vi "Waveform to CSV Converter.vi"(8 "error in (no error)":errorcluster, 11 "Waveform File Path (.wfm)":path) -> (0 "error out":errorcluster)   [LabVIEW 2013]
uses:
  <vilib>/Waveform/WDTFileIO.llb/Export Waveforms To Spreadsheet File (2D).vi
panel:
  out "Done":bool
  out "Zipping":bool
  out "Converting":bool
  out "Records read":i32
  # "Waveform to CSV Converter"
  # "This VI reads the Waveform data from the specified path and then writes all records to a CSV file.\nThis file is then added to a new Zip file and then deleted. The names of the CSV and Zip file are\nthe same as the Waveform file except with .wfm replaced with .csv and .zip respectively."
  # "27 Feb 2015\nby P. Lane"
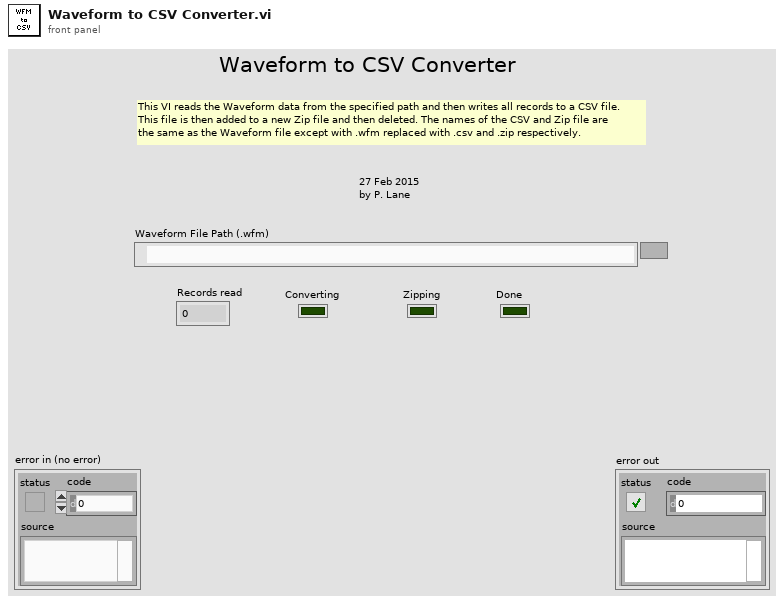
[diagram p1: front panel]
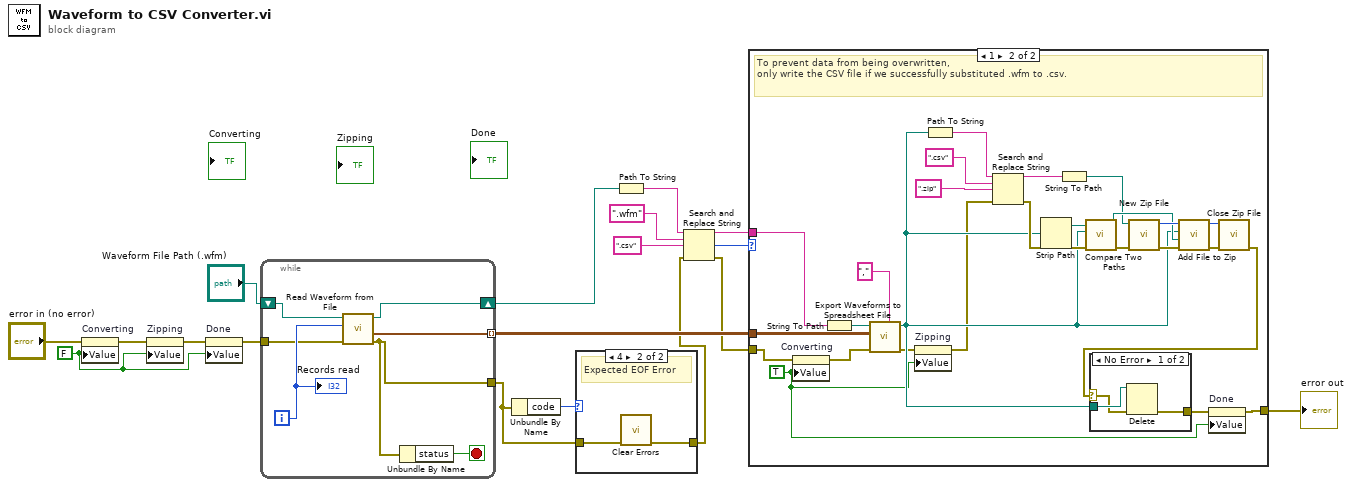
[diagram p0: block diagram]
diagram:
  w1 = FALSE ("Converted")
  n1 = property on="Converting" class="Bool (strict)"(error in="error in (no error)", "Value"=w1) -> (error out=w5:errorcluster)  [unwired: 1 in, 1 out]
  n2 = property on="Zipping" class="Bool (strict)"(error in=w5, "Value"=w1) -> (error out=w3:errorcluster)  [unwired: 1 in, 1 out]
  n3 = property on="Done" class="Bool (strict)"(error in=w3, "Value"=w1) -> (error out=w2:errorcluster)  [unwired: 1 in, 1 out]
  n4 = while {
    tunnel: [w23] -> w17 mode=indexing
    shift-right: [w22] -> w13
    shift-left: "Waveform File Path (.wfm)" -> [w21]
    tunnel: w2 -> [w20]
    tunnel: [w19] -> w9
    i -> [w25]
    stop <- w24 stop-if-true
    n5 = call <vilib>:"Read Waveform from File.vi"("error in (no error)"=w20, "offset (records:0)"=w25, "file path (dialog if empty)"=w21) -> ("error out"=w19:errorcluster, "all waveforms in record"=w23:waveform(dbl)[], "new file path (Not A Path if cancelled)"=w22:path)  [unwired: 3 in, 1 out]
    n6 = Unbundle By Name(w19) -> ("status"=w24:bool)
    "Records read" <- w25
  }
  n7 = Unbundle By Name(w9) -> ("code"=w10:i32)
  n8 = case shown="4" w10 {
    tunnel: w9 -> [w26 w28]
    tunnel: [w26 w27] -> w7
    frame 0, Default {
      # "Unexpected Error"
    }
    frame 4 {
      # "Expected EOF Error"
      n9 = call <vilib>:"Clear Errors.vi"("error in (no error)"=w28) -> ("error out"=w27:errorcluster)  [unwired: 6 in]
    }
  }
  n10 = Path To String(path=w13) -> (string=w14:string)
  n11 = Search and Replace String(input string=w14, search string=".wfm", replace string=".csv" ("replace string (\"\")"), error in=w7) -> (result string=w12:string, number of replacements=w11:i32, error out=w6:errorcluster)  [unwired: 4 in, 1 out]
  n12 = case shown="1" w11 {
    tunnel: w17 -> [_ w54]
    tunnel: w12 -> [_ w40]
    tunnel: w6 -> [w29 w37]
    tunnel: [w29 w31] -> w8
    frame 0, Default {
    }
    frame 1 {
      w30 = TRUE ("Converted")
      # "To prevent data from being overwritten,\nonly write the CSV file if we successfully substituted .wfm to .csv."
      n13 = property on="Converting" class="Bool (strict)"(error in=w37, "Value"=w30) -> (error out=w36:errorcluster)  [unwired: 1 in, 1 out]
      n14 = String To Path(string=w40) -> (path=w39:path)
      n15 = call-poly <vilib>:"Export Waveforms to Spreadsheet File.vi"("delimiter (Tab)"=",", "error in (no error)"=w36, "waveforms"=w54, "file path (dialog if empty)"=w39) -> ("error out"=w35:errorcluster, "new file path (Not A Path if cancelled)"=w38:path)  [unwired: 6 in]
      n16 = property on="Zipping" class="Bool (strict)"(error in=w35, "Value"=w30) -> (error out=w34:errorcluster)  [unwired: 1 in, 1 out]
      n17 = Path To String(path=w38) -> (string=w43:string)
      n18 = Search and Replace String(input string=w43, search string=".csv", replace string=".zip" ("replace string (\"\")"), error in=w34) -> (result string=w42:string, error out=w45:errorcluster)  [unwired: 4 in, 2 out]
      n19 = Strip Path(path=w38) -> (stripped path=w49:path)  [unwired: 1 out]
      n20 = String To Path(string=w42) -> (path=w41:path)
      n21 = call <vilib>:"Compare Two Paths.vi"("error in (no error)"=w45, "Path 2"=w38, "Path 1"=w49) -> ("error out"=w44:errorcluster, "Relative Path from 1 to 2"=w48:path)  [unwired: 5 in, 2 out]
      n22 = call <vilib>:"New Zip File.vi"("error in (no error)"=w44, "target"=w41) -> ("error out"=w52:errorcluster, "zip file out"=w53:i64)  [unwired: 3 in, 1 out]
      n23 = call <vilib>:"Add File to Zip.vi"("error in (no error)"=w52, "destination path in zip"=w48, "source file path"=w38, "zip file in"=w53) -> ("error out"=w50:errorcluster, "zip file out"=w51:i64)  [unwired: 6 in]
      n24 = call <vilib>:"Close Zip File.vi"("error in (no error)"=w50, "zip file in"=w51) -> ("error out"=w33:errorcluster)  [unwired: 5 in]
      n25 = case shown="No Error" w33 {
        selector: w33 -> [w57 w59]
        tunnel: w38 -> [w58 _]
        tunnel: [w56 w59] -> w32
        frame No Error {
          n26 = Delete(path (use dialog)=w58, error in=w57) -> (error out=w56:errorcluster)  [unwired: 3 in, 2 out]
        }
        frame Error {
        }
      }
      n27 = property on="Done" class="Bool (strict)"(error in=w32, "Value"=w30) -> (error out=w31:errorcluster)  [unwired: 1 in, 1 out]
    }
  }
  "error out" <- w8
